vi "FileIO_GetCurrentDateTimeString.vi"(11 "Error In":errorcluster) -> (8 "Date/Time String":string, 15 "Error Out":errorcluster)   [LabVIEW 2023]
doc: "Gets current date/time and formats to string in following format\n\nEX: [11_25_22_AM] [03_13_2015]"
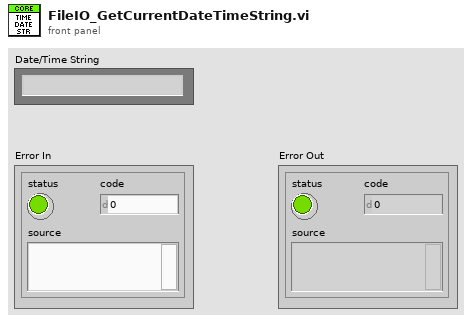
[diagram p1: front panel]
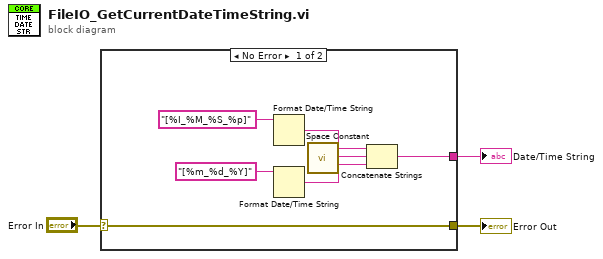
[diagram p0: block diagram]
diagram:
  n1 = case shown="No Error" "Error In" {
    selector: "Error In" -> [w4 w11]
    tunnel: [w8 _] -> w3
    tunnel: [w4 w11] -> w1
    frame No Error {
      n2 = Format Date/Time String(time format string (%c)="[%I_%M_%S_%p]") -> (date/time string=w6:string)  [unwired: 2 in]
      n3 = Format Date/Time String(time format string (%c)="[%m_%d_%Y]") -> (date/time string=w5:string)  [unwired: 2 in]
      n4 = call <vilib>:"Space Constant.vi"() -> ("String"=w7:string)
      n5 = Concatenate Strings(w6, w7, w5) -> (w8:string)
    }
    frame Error {
    }
  }
  "Date/Time String" <- w3
  "Error Out" <- w1
